vi "Draw coordinate reference.vi"(8 "error in (no error)":errorcluster, 10 "Details in":T1, 11 "Image in":T2) -> (0 "error out":errorcluster, 3 "Image out":T2)   [LabVIEW 2019]
uses:
  <vilib>/vision/Image Controls.llb/IMAQ Image.ctl
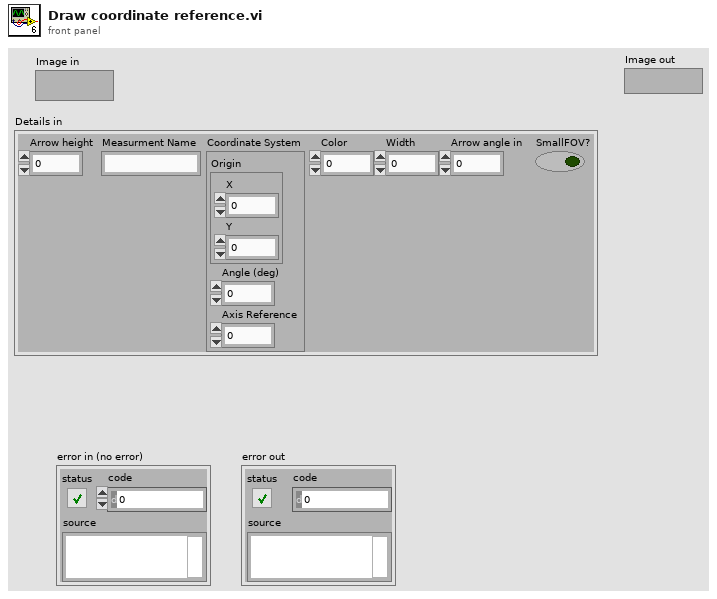
[diagram p1: front panel]
types:
  T1 = cluster{"Arrow height":dbl, "Measurment Name":string, "Coordinate System":cluster{"Origin":cluster{"X":sgl, "Y":sgl}, "Angle (deg)":sgl, "Axis Reference":u32}, "Color":u32, "Width":u32, "Arrow angle in":dbl, "SmallFOV?":bool}
  T2 = typedef "IMAQ Image.ctl" = refnum<image>
  T3 = enum16{"User-specified Font", "Application Font", "System Font", "Dialog Font"}
  T4 = cluster{"Desired Font (Application)":enum16{"User-specified Font", "Application Font", "System Font", "Dialog Font"}, "[User-specified Font]":cluster{"Font Name":string, "Size":i16, "Strikeout?":bool, "Italic?":bool, "Underline?":bool, "Outline?":bool, "Shadow?":bool, "Bold?":bool, "Rotation Angle":dbl}, "Horizontal Alignment":i16, "Vertical Alignment":i16}
  T5 = cluster{"Point 1":cluster{"x":dbl, "y":dbl}, "Point 2":cluster{"x":dbl, "y":dbl}}
  T6 = cluster{"Origin":cluster{"X":sgl, "Y":sgl}, "Angle (deg)":sgl, "Axis Reference":u32}
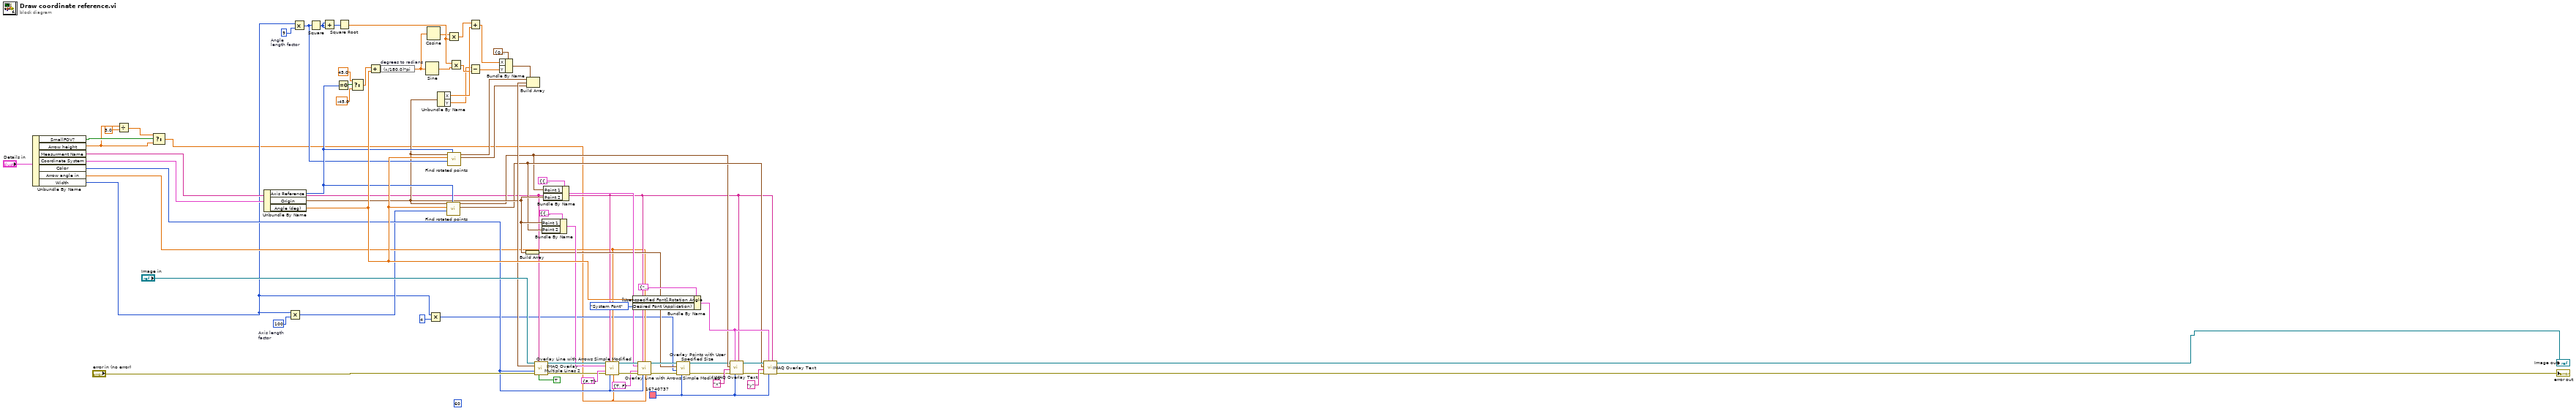
[diagram p0: block diagram]
diagram:
  w37 = u32 9  # Angle length factor
  w31 = u32 16740737 ("Color")
  (unwired) u32 60 ("Point Diameter (5)")
  w15 = u32 100  # Axis length factor
  n1 = Unbundle By Name("Details in") -> ("SmallFOV?"=w5:bool, "Arrow height"=w3:dbl, "Measurment Name"=w13:string, "Coordinate System"=w12:T6, "Color"=w11:u32, "Arrow angle in"=w10:dbl, "Width"=w6:u32)
  n2 = Divide(x=w3, y=3.0) -> (x/y=w1:dbl)
  n3 = Select(t=w1, s=w5, f=w3) -> (s? t:f=w2:dbl)
  n4 = Unbundle By Name(w12) -> ("Axis Reference"=w60:u32, "Origin"=w42:cluster{"X":sgl, "Y":sgl}, "Angle (deg)"=w71:sgl)
  n5 = Multiply(x=w6, y=w15) -> (x*y=w9:u32)
  n6 = Multiply(x=w6, y=w37) -> (x*y=w58:u32)
  n7 = Square(x=w58) -> (x^2=w56:u32)
  n8 = Add(x=w56, y=w56) -> (x+y=w57:u32)
  n9 = Equal To 0?(x=w60) -> (x = 0?=w61:bool)
  n10 = Square Root(x=w57) -> (sqrt(x)=w59:dbl)
  n11 = Select(t=sgl 45.0 ("Angle (deg)"), s=w61, f=sgl -45.0 ("Angle (deg)")) -> (s? t:f=w72:sgl)
  n12 = Add(x=w72, y=w71) -> (x+y=w38:sgl)
  n13 = expression code="(x/180.0)*pi" "degrees to radians"(w38) -> (w39:sgl)
  n14 = Sine(x=w39) -> (sin(x)=w41:sgl)
  n15 = Cosine(x=w39) -> (cos(x)=w40:sgl)
  n16 = Multiply(x=w6, y=u32 4) -> (x*y=w7:u32)
  n17 = Unbundle By Name(w42) -> ("X"=w69:sgl, "Y"=w54:sgl)
  n18 = call "Find rotated points.vi"("Axis reference"=w60, "Line seg \nlength"=w9, "Angle (deg)"=w71, "Origin"=w42) -> ("Point Coordinates (y axis)"=w26:cluster{"X":dbl, "Y":dbl}, "Point 1 coordinates (x axis)"=w25:cluster{"X":dbl, "Y":dbl})  [unwired: 6 in]
  n19 = Multiply(x=w40, y=w59) -> (x*y=w68:dbl)
  n20 = call "Find rotated points.vi"("Axis reference"=w60, "Line seg \nlength"=w58, "Angle (deg)"=w71, "Origin"=w42) -> ("Point Coordinates (y axis)"=w47:cluster{"X":dbl, "Y":dbl}, "Point 1 coordinates (x axis)"=w45:cluster{"X":dbl, "Y":dbl})  [unwired: 6 in]
  n21 = Multiply(x=w59, y=w41) -> (x*y=w55:dbl)
  n22 = Add(x=w68, y=w69) -> (x+y=w70:dbl)
  n23 = Subtract(x=w54, y=w55) -> (x-y=w44:dbl)
  n24 = Bundle By Name(cluster=cluster{"X":sgl, "Y":sgl} {"X"=0.0, "Y"=0.0} ("Coordinate System.Origin"), "X"=w70, "Y"=w44) -> (w46:cluster{"X":sgl, "Y":sgl})
  n25 = Build Array(w42) -> (w16:cluster{"X":sgl, "Y":sgl}[])
  n26 = Build Array(w45, w46, w47) -> (w48:cluster{"X":dbl, "Y":dbl}[])
  n27 = call "IMAQ Overlay Multiple Lines 2"("Image"="Image in", "Group"=w13, "Line End Points"=w48, "Color"=w11, "error in (no error)"="error in (no error)", "Maintain Width?"=TRUE) -> ("Image Out"=w53:T2, "error out"=w51:errorcluster)  [unwired: 8 in]
  n28 = Bundle By Name(cluster=T5 {"Point 1"={"x"=0.0, "y"=0.0}, "Point 2"={"x"=0.0, "y"=0.0}} ("Line Coordinates"), "Point 1"=w42, "Point 2"=w26) -> (w21:T5)
  n29 = Bundle By Name(cluster=T5 {"Point 1"={"x"=0.0, "y"=0.0}, "Point 2"={"x"=0.0, "y"=0.0}} ("Line Coordinates"), "Point 1"=w25, "Point 2"=w42) -> (w20:T5)
  n30 = call "Overlay Line with Arrows Simple Modified.vi"("Image In"=w53, "Group"=w13, "Angle Coefficient"=w10, "Line Coordinates"=w21, "Arrows"=cluster{"Start point":bool, "End point":bool} {"Start point"=FALSE, "End point"=TRUE}, "error in"=w51, "Color"=w11, "Height Coefficient"=w2) -> ("Image Out"=w66:T2, "error out"=w67:errorcluster)  [unwired: 6 in]
  n31 = Bundle By Name(cluster=T4 {"Desired Font (Application)"=enum."Application Font", "[User-specified Font]"={"Font Name"="", "Size"=12, "Strikeout?"=FALSE, "Italic?"=FALSE, "Underline?"=FALSE, "Outline?"=FALSE, "Shadow?"=FALSE, "Bold?"=FALSE, "Rotation Angle"=0.0}, "Horizontal Alignment"=0, "Vertical Alignment"=0} ("Font, Size & Style"), "[User-specified Font].Rotation Angle"=w71, "Desired Font (Application)"=T3."System Font") -> (w29:T4)
  n32 = call "Overlay Line with Arrows Simple Modified.vi"("Image In"=w66, "Group"=w13, "Angle Coefficient"=w10, "Line Coordinates"=w20, "Arrows"=cluster{"Start point":bool, "End point":bool} {"Start point"=TRUE, "End point"=FALSE}, "error in"=w67, "Color"=w11, "Height Coefficient"=w2) -> ("Image Out"=w22:T2, "error out"=w17:errorcluster)  [unwired: 6 in]
  n33 = call "Overlay Points with User Specified Size.vi"("Color"=w31, "error in"=w17, "Point Diameter (5)"=w7, "Points"=w16, "Image In"=w22) -> ("error out"=w24:errorcluster, "Image Out"=w23:T2)  [unwired: 5 in]
  n34 = call "IMAQ Overlay Text"("Group"=w13, "Text Color (black)"=w31, "Font, Size & Style"=w29, "error in (no error)"=w24, "String"="x", "Origin"=w25, "Image"=w23) -> ("error out"=w32:errorcluster, "Image Out"=w27:T2)  [unwired: 3 in]
  n35 = call "IMAQ Overlay Text"("Group"=w13, "Text Color (black)"=w31, "Font, Size & Style"=w29, "error in (no error)"=w32, "String"="y", "Origin"=w26, "Image"=w27) -> ("error out"=→"error out":errorcluster, "Image Out"=→"Image out":T2)  [unwired: 3 in]
